vi "UPDGetData(HandCalib).vi"() -> ()   [LabVIEW 2017]
panel:
  out "Calibrated":T1={"head"={"orientation"={"roll"=0.41476414789520294, "pitch"=-9.61807061952259, "yaw"=51.632320891332185}, "position"={"x"=0.704318, "y"=0.128604, "z"=-0.985214}}, "hands"={"left"={"position"={"x"=nan, "y"=nan, "z"=nan}}, "right"={"position"={"x"=0.0, "y"=0.0, "z"=0.0}}}, "buttons"={"a"=0, "b"=0, "x"=0, "y"=0}}
  out "Raw":T1={"head"={"orientation"={"roll"=0.007239, "pitch"=-0.167867, "yaw"=-0.901154}, "position"={"x"=0.704318, "y"=0.128604, "z"=-0.985214}}, "hands"={"left"={"position"={"x"=0.507599, "y"=-0.151934, "z"=-0.712968}}, "right"={"position"={"x"=0.857917, "y"=0.158242, "z"=-0.84482}}}, "buttons"={"a"=0, "b"=0, "x"=0, "y"=0}}
  in  "stop":bool
  in  "Arm X Min":dbl
  in  "Arm X Max":dbl=100.0
  in  "error in (no error)":errorcluster
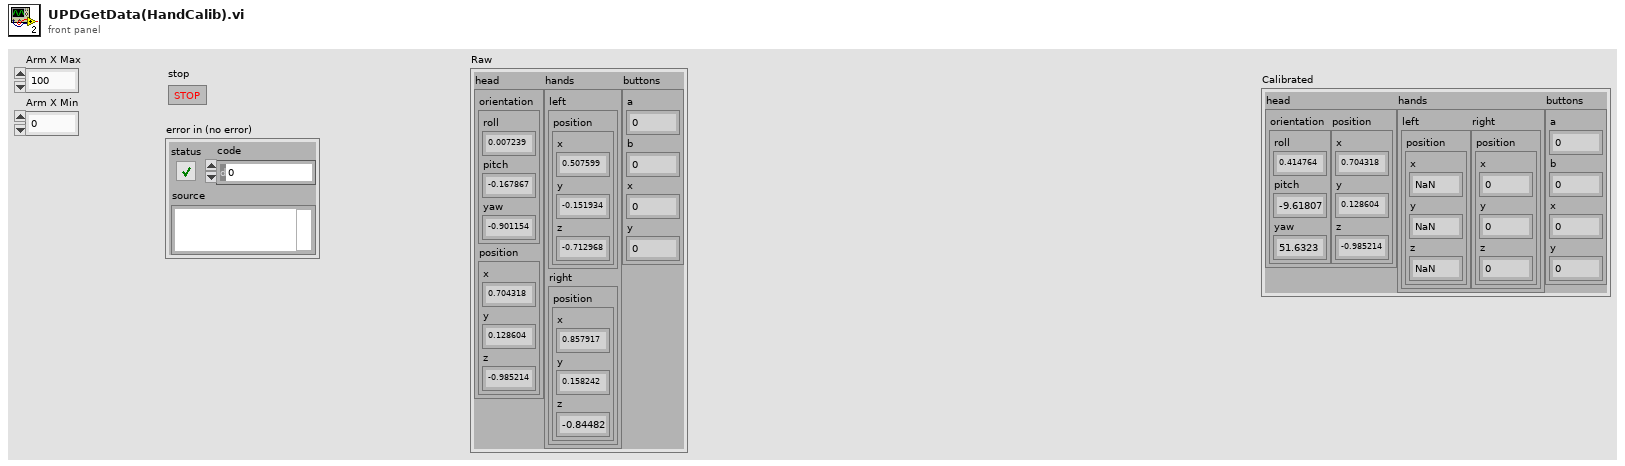
[diagram p1: front panel]
types:
  T1 = cluster{"head":cluster{"orientation":cluster{"roll":dbl, "pitch":dbl, "yaw":dbl}, "position":cluster{"x":dbl, "y":dbl, "z":dbl}}, "hands":cluster{"left":cluster{"position":cluster{"x":dbl, "y":dbl, "z":dbl}}, "right":cluster{"position":cluster{"x":dbl, "y":dbl, "z":dbl}}}, "buttons":cluster{"a":i32, "b":i32, "x":i32, "y":i32}}
  T2 = enum16{"Calibrate", "RightMax", "RightMin", "LeftMax", "LeftMin"}
  T3 = cluster{"head":cluster{"orientation":cluster{"roll":dbl, "pitch":dbl, "yaw":dbl}, "position":cluster{"x":dbl, "y":dbl, "z":dbl}}, "hands":cluster{"left":cluster{"position":cluster{"x":dbl, "y":dbl, "z":dbl}, "orientation":cluster{"roll":dbl, "pitch":dbl, "yaw":dbl}}, "right":cluster{"position":cluster{"x":dbl, "y":dbl, "z":dbl}, "orientation":cluster{"roll":dbl, "pitch":dbl, "yaw":dbl}}}, "buttons":cluster{"a":i32, "b":i32, "x":i32, "y":i32, "leftTrig":dbl, "rightTrig":dbl, "left_jstick":cluster{"x":dbl, "y":dbl}, "right_jstick":cluster{"x":dbl, "y":dbl}}}
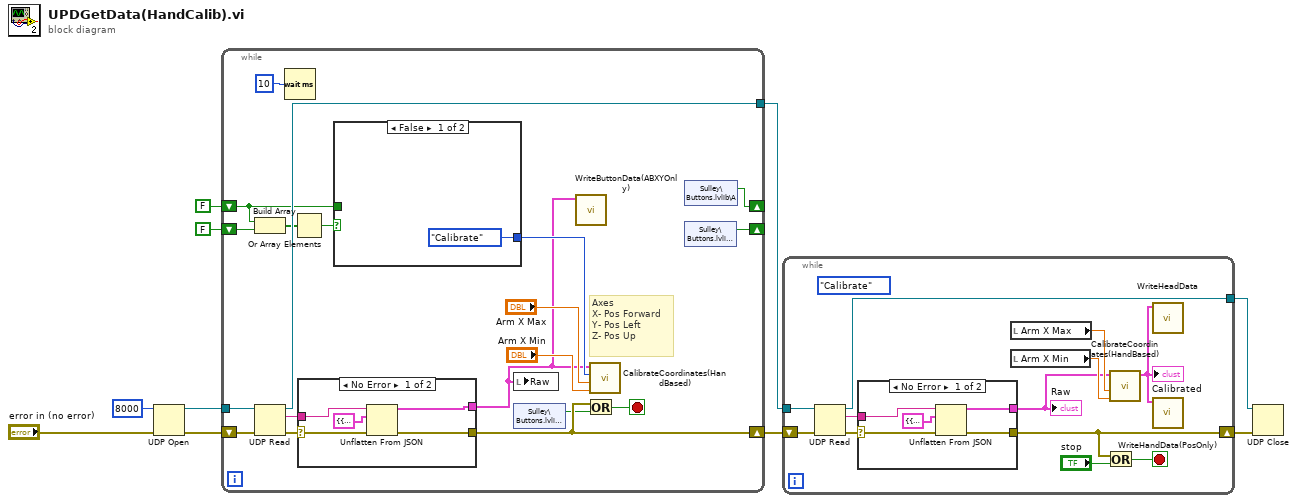
[diagram p0: block diagram]
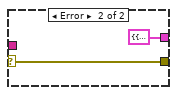
[diagram p2: hidden frame]
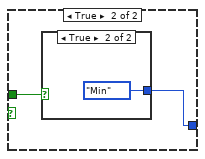
[diagram p3: hidden frame]
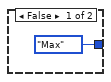
[diagram p4: hidden frame]
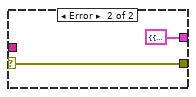
[diagram p5: hidden frame]
diagram:
  n1 = UDP Open(8:"error in (no error)", 11:8000) -> (port=w8:refnum<k16>, 0:w9:errorcluster)  [unwired: 3 in, 1 out]
  n2 = while {
    tunnel: w8 -> [w28]
    tunnel: [w27] -> w4
    shift-right: [w22] -> w6
    shift-left: w9 -> [w29]
    shift-right: [w15] -> _
    shift-left: FALSE ("Boolean") -> [w12]
    shift-right: [w14] -> _
    shift-left: FALSE ("Boolean") -> [w13]
    stop <- w23 stop-if-true
    # "Axes\nX- Pos Forward\nY- Pos Left\nZ- Pos Up"
    n3 = Build Array(w12, w13) -> (w19:bool[])
    n4 = UDP Read(connection ID=w28, 8:w29) -> (data out=w25:string, error out=w26:errorcluster, 3:w27:refnum<k16>)  [unwired: 2 in, 2 out]
    n5 = Wait (ms)(milliseconds to wait=u32 10) -> ()  [unwired: 1 out]
    n6 = Or Array Elements(Boolean array=w19) -> (logical OR=w18:bool)
    n7 = case shown="No Error" w26 {
      selector: w26 -> [w39 w41]
      tunnel: [w38 w41] -> w22
      tunnel: w25 -> [w37 _]
      tunnel: [w36 T1 {"head"={"orientation"={"roll"=0.0, "pitch"=0.0, "yaw"=0.0}, "position"={"x"=0.0, "y"=0.0, "z"=0.0}}, "hands"={"left"={"position"={"x"=0.0, "y"=0.0, "z"=0.0}}, "right"={"position"={"x"=0.0, "y"=0.0, "z"=0.0}}}, "buttons"={"a"=0, "b"=0, "x"=0, "y"=0}}] -> w11
      frame No Error {
        n8 = Unflatten From JSON(JSON string=w37, type and defaults=T1 {"head"={"orientation"={"roll"=0.0, "pitch"=0.0, "yaw"=0.0}, "position"={"x"=0.0, "y"=0.0, "z"=0.0}}, "hands"={"left"={"position"={"x"=0.0, "y"=0.0, "z"=0.0}}, "right"={"position"={"x"=0.0, "y"=0.0, "z"=0.0}}}, "buttons"={"a"=0, "b"=0, "x"=0, "y"=0}}, error in (no error)=w39) -> (value=w36:T1, error out=w38:errorcluster)  [unwired: 4 in]
      }
      frame Error {
      }
    }
    n9 = case shown="False" w18 {
      tunnel: [enum16{"Calibrate", "Max", "Min"}."Calibrate" ("Control") w31] -> w17
      tunnel: w12 -> [_ w32]
      frame False {
      }
      frame True {
        n10 = case shown="True" w32 {
          tunnel: [enum16{"Calibrate", "Max", "Min"}."Max" ("Control") enum16{"Calibrate", "Max", "Min"}."Min" ("Control")] -> w31
          frame False {
          }
          frame True {
          }
        }
      }
    }
    n11 = local write "Raw"(w11) -> ()
    n12 = shared-variable "Sulley\\Buttons.lvlib\\X"() -> (w16:bool)  [unwired: 1 in, 1 out]
    n13 = call "WriteButtonData(ABXYOnly).vi"("Cluster"=w11) -> ()  [unwired: 11 in]
    n14 = Or(x=w22, y=w16) -> (x .or. y?=w23:bool)
    n15 = call "CalibrateCoordinates(HandBased).vi"("Arm X Min"="Arm X Min", "Arm X Max"="Arm X Max", "Control"=w17, "Cluster"=w11) -> ()  [unwired: 6 in, 2 out]
    n16 = shared-variable "Sulley\\Buttons.lvlib\\A"() -> (w15:bool)  [unwired: 1 in, 1 out]
    n17 = shared-variable "Sulley\\Buttons.lvlib\\B"() -> (w14:bool)  [unwired: 1 in, 1 out]
  }
  n18 = while {
    shift-right: [w49] -> w5
    shift-left: w6 -> [w50]
    tunnel: w4 -> [w51]
    tunnel: [w47] -> w3
    stop <- w48 stop-if-true
    (unwired) T2."Calibrate" ("Control")
    n19 = UDP Read(connection ID=w51, 8:w50) -> (data out=w52:string, error out=w53:errorcluster, 3:w47:refnum<k16>)  [unwired: 2 in, 2 out]
    n20 = case shown="No Error" w53 {
      selector: w53 -> [w58 w60]
      tunnel: [w57 w60] -> w49
      tunnel: w52 -> [w56 _]
      tunnel: [w54 T1 {"head"={"orientation"={"roll"=0.0, "pitch"=0.0, "yaw"=0.0}, "position"={"x"=0.0, "y"=0.0, "z"=0.0}}, "hands"={"left"={"position"={"x"=0.0, "y"=0.0, "z"=0.0}}, "right"={"position"={"x"=0.0, "y"=0.0, "z"=0.0}}}, "buttons"={"a"=0, "b"=0, "x"=0, "y"=0}}] -> w42
      frame No Error {
        n21 = Unflatten From JSON(JSON string=w56, type and defaults=T1 {"head"={"orientation"={"roll"=0.0, "pitch"=0.0, "yaw"=0.0}, "position"={"x"=0.0, "y"=0.0, "z"=0.0}}, "hands"={"left"={"position"={"x"=0.0, "y"=0.0, "z"=0.0}}, "right"={"position"={"x"=0.0, "y"=0.0, "z"=0.0}}}, "buttons"={"a"=0, "b"=0, "x"=0, "y"=0}}, error in (no error)=w58) -> (value=w54:T1, error out=w57:errorcluster)  [unwired: 4 in]
      }
      frame Error {
      }
    }
    "Raw" <- w42
    n22 = local read "Arm X Max"() -> (w44:dbl)
    n23 = local read "Arm X Min"() -> (w45:dbl)
    n24 = Or(x=w49, y="stop") -> (x .or. y?=w48:bool)
    n25 = call "CalibrateCoordinates(HandBased).vi"("Arm X Min"=w45, "Arm X Max"=w44, "Cluster"=w42) -> ("Calibrated"=w46:T3)  [unwired: 7 in, 1 out]
    "Calibrated" <- w46
    n26 = call "WriteHeadData.vi"("Cluster"=w46) -> ()  [unwired: 11 in]
    n27 = call "WriteHandData(PosOnly).vi"("Cluster"=w46) -> ()  [unwired: 11 in]
  }
  n28 = UDP Close(connection ID=w3, 8:w5) -> ()  [unwired: 2 out]
